vi "Measure.vi"(7 "New Integration Time":i32, 8 "error in (no error)":errorcluster, 11 "EpiWrapper in":refnum<class "EpiWrapper.lvclass">) -> (0 "error out":errorcluster, 2 "Data Out":T1 {"50mA Data"."Current,mA" format="%_6g"; "50mA Data"."WL" format="%_6g"; "50mA Data"."Voltage" format="%_6g"; "50mA Data"."Power" format="%_6g"; "20mA Data"."Reverse" format="%#_3g"; "20mA Data"."Current,mA" format="%_6g"; "20mA Data"."Knee Current" format="%#_3g"; "20mA Data"."WL" format="%_6g"; "20mA Data"."Voltage" format="%_6g"; "20mA Data"."Power" format="%_5g"}, 3 "EpiWrapper out":refnum<class "EpiWrapper.lvclass">, 4 "ExcelOut":string, 5 "ReMeasure?":bool)   [LabVIEW 2012, in "EpiWrapper.lvclass"]
uses:
  EpiWrapper.lvclass
  Controls/TestData.ctl
  EpiWrapper.lvclass/EpiWrapper.ctl
  Instruments.lvclass
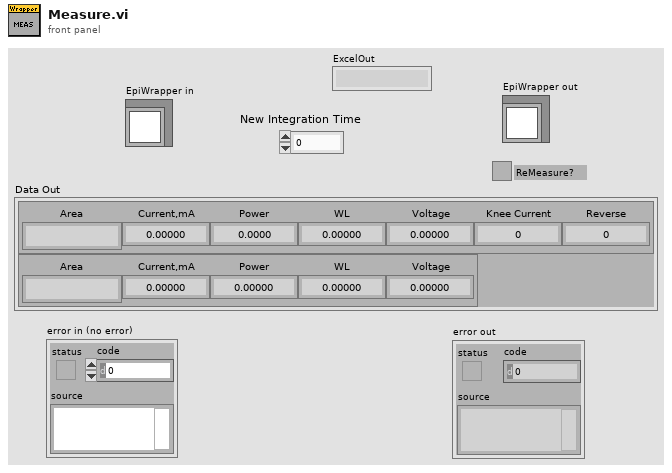
[diagram p1: front panel]
types:
  T1 = typedef "TestData.ctl" = cluster{"20mA Data":cluster{"Area":string, "Current,mA":dbl, "Power":dbl, "WL":dbl, "Voltage":dbl, "Knee Current":dbl, "Reverse":dbl}, "50mA Data":cluster{"Area":string, "Current,mA":dbl, "Power":dbl, "WL":dbl, "Voltage":dbl}}
  T2 = cluster{"Area":string, "Current,mA":dbl, "Power":dbl, "WL":dbl, "Voltage":dbl, "Knee Current":dbl, "Reverse":dbl}
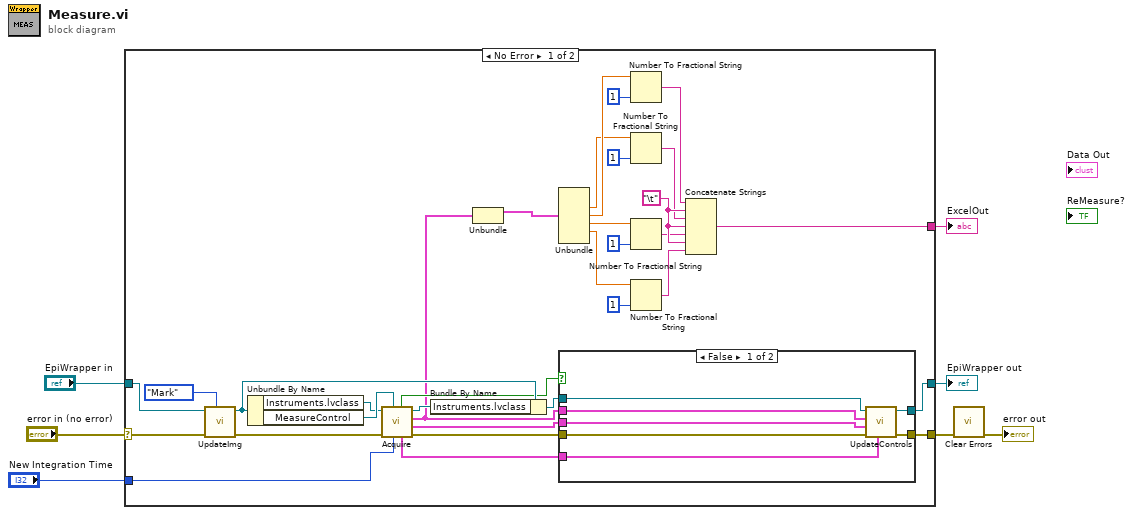
[diagram p0: block diagram]
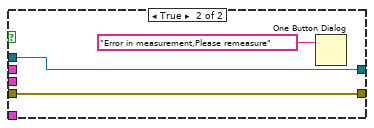
[diagram p2: hidden frame]
diagram:
  n1 = case shown="No Error" "error in (no error)" {
    selector: "error in (no error)" -> [w39 w51]
    tunnel: [w28 w51] -> w3
    tunnel: [w29 w50] -> w5
    tunnel: "EpiWrapper in" -> [w34 w50]
    tunnel: "New Integration Time" -> [w26 _]
    tunnel: [w13 _] -> w1
    frame No Error {
      w21 = "\t"
      n2 = call-dynamic "UpdateImg.vi"("Enum"=enum16{"Mark", "Clear All"}."Mark", "error in (no error)"=w39, "EpiWrapper in"=w34) -> ("error out"=w38:errorcluster, "EpiWrapper out"=w33:refnum<class "EpiWrapper.lvclass">)  [unwired: 7 in]
      n3 = Unbundle By Name(w33) -> ("Instruments.lvclass"=w36:refnum<class "Instruments.lvclass">, "MeasureControl"=w37:refnum<vi>)
      n4 = call-dynamic "Acquire.vi"("Integration Time"=w26, "MeasureControl"=w37, "error in (no error)"=w38, "Instruments in"=w36) -> ("error out"=w27:errorcluster, "20mA Spectra"=w25:cluster{"Wavelength":dbl[], "EL Spectrum":dbl[]}, "Data Out"=w24:T1, "Instruments out"=w35:refnum<class "Instruments.lvclass">, "50mA Spectra"=w8:cluster{"Wavelength":dbl[], "EL Spectrum":dbl[]}, "Overrange"=w30:bool)  [unwired: 2 in]
      n5 = Bundle By Name(cluster=w33, "Instruments.lvclass"=w35) -> (w31:refnum<class "EpiWrapper.lvclass">)
      n6 = Unbundle(w24) -> ("20mA Data"=w23:T2)  [unwired: 1 out]
      n7 = Unbundle(w23) -> ("Power"=w19:dbl, "WL"=w22:dbl, "Voltage"=w18:dbl, "Knee Current"=w17:dbl)  [unwired: 3 out]
      n8 = case shown="False" w30 {
        tunnel: w24 -> [w46 _]
        tunnel: w31 -> [w45 w47]
        tunnel: [w44 w47] -> w29
        tunnel: [w43 w48] -> w28
        tunnel: w27 -> [w42 w48]
        tunnel: w25 -> [w41 _]
        tunnel: w8 -> [w40 _]
        frame False {
          n9 = call-dynamic "UpdateControls.vi"("50mA Spectra"=w40, "error in (no error)"=w42, "20mA Spectra"=w41, "Data In"=w46, "EpiWrapper in"=w45) -> ("error out"=w43:errorcluster, "EpiWrapper out"=w44:refnum<class "EpiWrapper.lvclass">)  [unwired: 5 in]
        }
        frame True {
          n10 = One Button Dialog(message="Error in measurement,Please remeasure") -> ()  [unwired: 1 in, 1 out]
        }
      }
      n11 = Number To Fractional String(number=w22, precision (6)=i16 1) -> (F-format string=w20:string)  [unwired: 2 in]
      n12 = Number To Fractional String(number=w19, precision (6)=i16 1) -> (F-format string=w16:string)  [unwired: 2 in]
      n13 = Number To Fractional String(number=w18, precision (6)=i16 1) -> (F-format string=w15:string)  [unwired: 2 in]
      n14 = Number To Fractional String(number=w17, precision (6)=i16 1) -> (F-format string=w14:string)  [unwired: 2 in]
      n15 = Concatenate Strings(w20, w21, w16, w21, w15, w21, w14) -> (w13:string)
    }
    frame Error {
    }
  }
  "EpiWrapper out" <- w5
  "ExcelOut" <- w1
  n16 = call <vilib>:"Clear Errors.vi"("error in (no error)"=w3) -> ("error out"=→"error out":errorcluster)  [unwired: 6 in]
